vi "Read Limit Test Result.vi"(7 "Limit Test Data Size (0)":i32, 8 "error in (no error)":errorcluster, 9 "Limit Test Data Offset (0)":i32, 10 "Channel (1: Channel 1)":i32(ring)=1 items=["Channel 1"=1, "Channel 2"=2], 11 "VISA resource name":refnum<visa-resource-name>) -> (0 "error out":errorcluster, 2 "Limit Test Data":T1, 3 "VISA resource name out":refnum<visa-resource-name>, 5 "Limit Test Failed?":bool[](array[boolean]))   [LabVIEW 2012, in "Keysight B2980 Series.lvlib"]
doc: "Returns limit test data."
uses:
  Keysight B2980 Series.lvlib
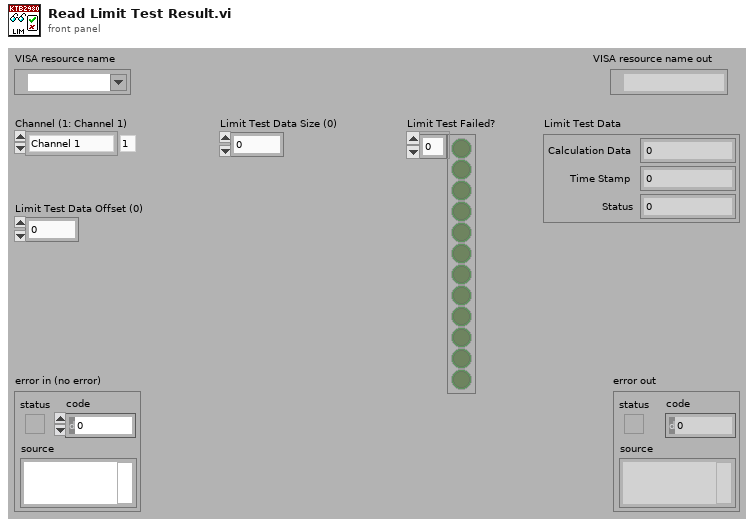
[diagram p1: front panel]
types:
  T1 = cluster{"Calculation Data":dbl, "Time Stamp":dbl, "Status":dbl}
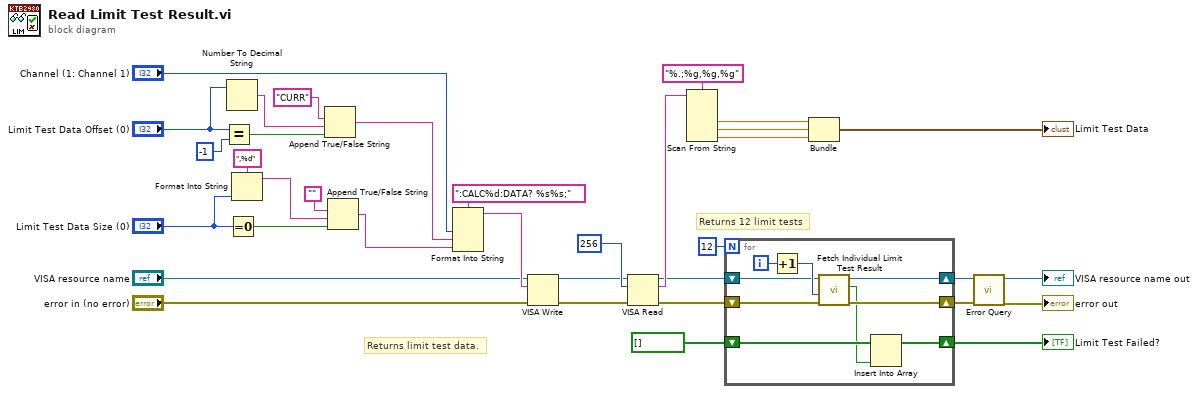
[diagram p0: block diagram]
diagram:
  # "Returns 12 limit tests"
  # "Returns limit test data."
  n1 = Equal?(x="Limit Test Data Offset (0)", y=-1) -> (x = y?=w10:bool)
  n2 = Number To Decimal String(number="Limit Test Data Offset (0)") -> (decimal integer string=w7:string)  [unwired: 1 out]
  n3 = Equal To 0?(x="Limit Test Data Size (0)") -> (x = 0?=w6:bool)
  n4 = Format Into String(format string=",%d", "Limit Test Data Size (0)") -> (resulting string=w4:string)  [unwired: 2 in, 1 out]
  n5 = Append True/False String(1:w10, 2:w7, 3:"CURR") -> (0:w8:string)  [unwired: 1 in]
  n6 = Append True/False String(1:w6, 2:w4, 3:"") -> (0:w3:string)  [unwired: 1 in]
  n7 = Format Into String(format string=":CALC%d:DATA? %s%s;", "Channel (1: Channel 1)", w8, w3) -> (resulting string=w34:string)  [unwired: 2 in, 1 out]
  n8 = VISA Write(VISA resource name="VISA resource name", write buffer=w34, error in (no error)="error in (no error)") -> (VISA resource name out=w30:refnum<visa-resource-name>, error out=w29:errorcluster)  [unwired: 1 out]
  n9 = VISA Read(VISA resource name=w30, byte count=u32 256, error in (no error)=w29) -> (VISA resource name out=w19:refnum<visa-resource-name>, read buffer=w26:string, error out=w18:errorcluster)  [unwired: 1 out]
  n10 = Scan From String(format string="%.;%g,%g,%g", input string=w26) -> (output 1=w24:dbl, output 2=w23:dbl, output 3=w22:dbl)  [unwired: 2 in, 6 out]
  n11 = for {
    N: 12 -> [_]
    shift-right: [w40] -> w15
    shift-left: w19 -> [w42]
    shift-right: [w39] -> w14
    shift-left: w18 -> [w41]
    shift-right: [w36] -> w13
    shift-left: bool[] [] ("Limit Test Failed?") -> [w38]
    i -> [w44]
    n12 = Increment(x=w44) -> (x+1=w43:i32)
    n13 = call "Fetch Individual Limit Test Result.vi"("error in (no error)"=w41, "Limit Test Number (1)"=w43, "VISA resource name"=w42) -> ("error out"=w39:errorcluster, "Limit Test Failed"=w37:bool, "VISA resource name out"=w40:refnum<visa-resource-name>)  [unwired: 1 in, 5 out]
    n14 = Insert Into Array(array=w38, new element=w37) -> (w36:bool[])  [unwired: 1 in]
  }
  "Limit Test Failed?" <- w13
  n15 = Bundle(w24, w23, w22) -> (→"Limit Test Data":cluster{dbl, dbl, dbl})  [unwired: 1 out]
  n16 = call "Error Query.vi"("error in (no error)"=w14, "VISA resource name"=w15) -> ("error out"=→"error out":errorcluster, "VISA resource name out"=→"VISA resource name out":refnum<visa-resource-name>)  [unwired: 8 out]
